vi "referenceToValue.vi"(8 "Error In":errorcluster, 11 "Reference Array":refnum<vi>[](array[refnum])) -> (0 "Error Out":errorcluster, 3 "Value Out Cluster":T1)   [LabVIEW 2018]
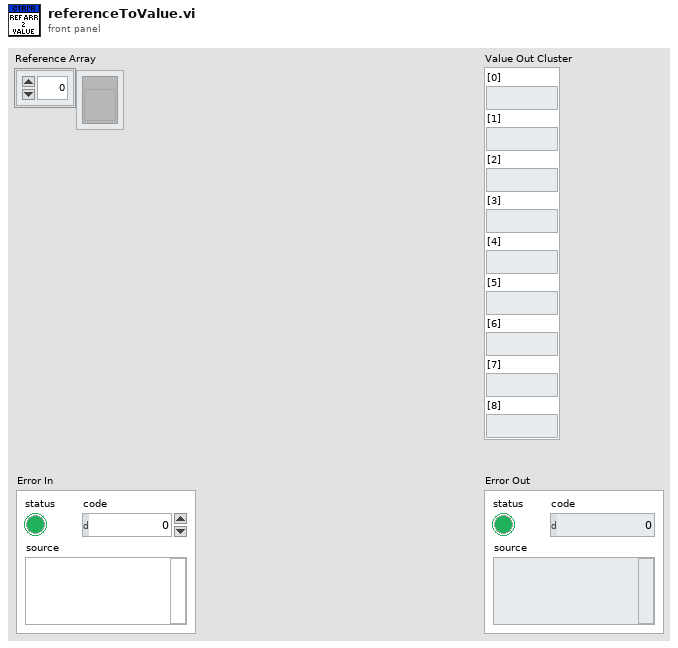
[diagram p1: front panel]
types:
  T1 = cluster{"[0]":string, "[1]":string, "[2]":string, "[3]":string, "[4]":string, "[5]":string, "[6]":string, "[7]":string, "[8]":string}
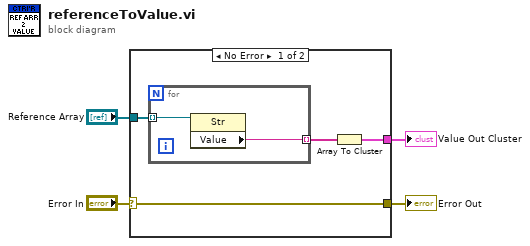
[diagram p0: block diagram]
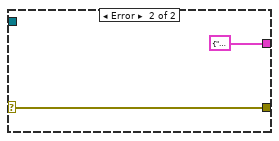
[diagram p2: hidden frame]
diagram:
  n1 = case shown="No Error" "Error In" {
    selector: "Error In" -> [w5 w11]
    tunnel: [w8 T1 {"[0]"="", "[1]"="", "[2]"="", "[3]"="", "[4]"="", "[5]"="", "[6]"="", "[7]"="", "[8]"=""}] -> w4
    tunnel: "Reference Array" -> [w6 _]
    tunnel: [w5 w11] -> w1
    frame No Error {
      n2 = for {
        tunnel: w6 -> [w10] mode=indexing
        tunnel: [w9] -> w7 mode=indexing
        n3 = property class="Str"(reference=w10) -> ("Value"=w9:string)  [unwired: 1 in, 2 out]
      }
      n4 = Array To Cluster(array=w7) -> (cluster=w8:T1)
    }
    frame Error {
    }
  }
  "Value Out Cluster" <- w4
  "Error Out" <- w1
